vi "Globales.vi"() -> ()   [LabVIEW 2019]
panel:
  in  "CNT90_Detenido":bool
  in  "K2002_Detenido":bool
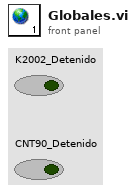
[diagram p1: front panel]
diagram:
